vi "Check Refnum Class.vi"(8 "error in (no error)":errorcluster, 11 "Numeric Field in":refnum<class "Numeric Field.lvclass">) -> (0 "error out":errorcluster, 3 "Numeric Field out":refnum<class "Numeric Field.lvclass">)   [LabVIEW 2020, in "Numeric Field.lvclass"]
uses:
  Numeric Field.lvclass
  C:/Users/User/Desktop/Raman Program/Database OOP/source/Field/Field.lvclass
  Field/Field.lvclass/Field.ctl
  Field/Field.lvclass
panel:
  # "For override: make sure that the wired control refnum class matches the field child class"
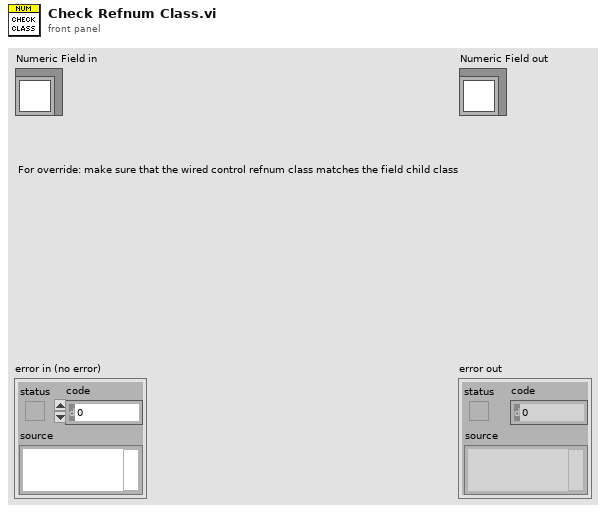
[diagram p1: front panel]
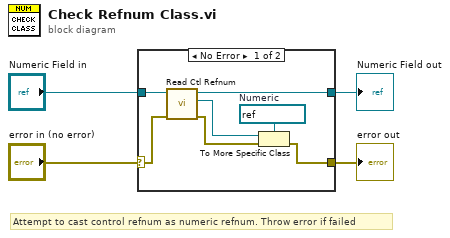
[diagram p0: block diagram]
diagram:
  # "Attempt to cast control refnum as numeric refnum. Throw error if failed"
  n1 = case shown="No Error" "error in (no error)" {
    selector: "error in (no error)" -> [w9 w12]
    tunnel: "Numeric Field in" -> [w11 w13]
    tunnel: [w10 w13] -> w2
    tunnel: [w5 w12] -> w1
    frame No Error {
      w6 = refnum<vi> refnum  # Numeric
      n2 = call "Read Ctl Refnum.vi"("error in (no error)"=w9, "Field in"=w11) -> ("error out"=w8:errorcluster, "Ctl Refnum"=w7:refnum<vi>, "Field out"=w10:refnum<class "Numeric Field.lvclass">)  [unwired: 7 in]
      n3 = To More Specific Class(target class=w6, reference=w7, error in=w8) -> (error out=w5:errorcluster)  [unwired: 1 out]
    }
    frame Error {
    }
  }
  "error out" <- w1
  "Numeric Field out" <- w2
